vi "Reset.vi"(8 "error in (no error)":errorcluster, 10 "target time(s)":dbl, 11 "Timer in":refnum<class "Timer.lvclass">) -> (0 "error out":errorcluster, 3 "Timer out":refnum<class "Timer.lvclass">)   [LabVIEW 2020, in "Timer.lvclass"]
uses:
  Timer.lvclass
  Timer.lvclass/Timer.ctl
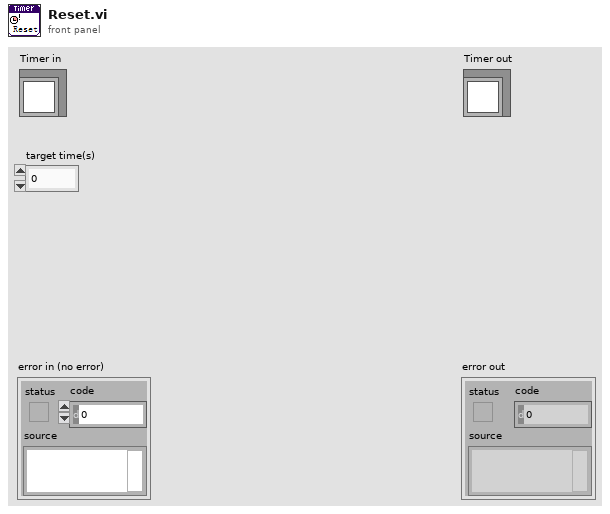
[diagram p1: front panel]
types:
  T1 = cluster{"target time(ms)":u32, "elapsed time(ms)":u32, "start time":u32, "pause":bool}
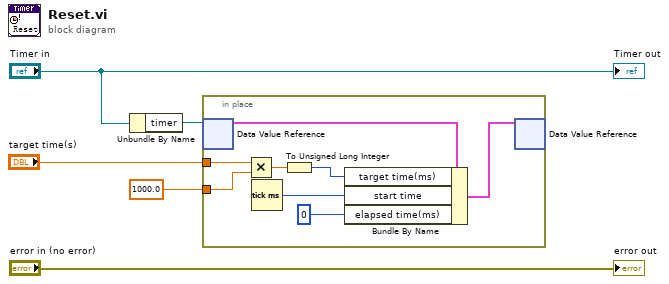
[diagram p0: block diagram]
diagram:
  n1 = Unbundle By Name("Timer in") -> ("timer"=w2:refnum<data-value>)
  n2 = in-place {
    in-place-border: "target time(s)" -> [w11]
    in-place-border: 1000.0 ("y") -> [w8]
    n3 = in-place-dvr #1(w2) -> (w10:T1)  [unwired: 1 out]
    n4 = Multiply(x=w11, y=w8) -> (x*y=w12:dbl)
    n5 = Tick Count (ms)() -> (millisecond timer value=w13:u32)
    n6 = To Unsigned Long Integer(number=w12) -> (unsigned 32bit integer=w7:u32)
    n7 = Bundle By Name(cluster=w10, "target time(ms)"=w7, "start time"=w13, "elapsed time(ms)"=u32 0) -> (w9:T1)
    n8 = in-place-dvr #1(w9) -> ()  [unwired: 2 out]
  }
  "error out" <- "error in (no error)"
  "Timer out" <- "Timer in"
